vi "testMove.vi"() -> ()   [LabVIEW 2019]
uses:
  WSCbot_V3_Toolkit.lvlibp
panel:
  out "ENC (deg) 2":dbl[](array[numeric])
  in  "Enable?":bool=TRUE
  out "ENC (deg)":dbl[](array[numeric])
  in  "4xMotor(deg/s)":dbl[](array[numeric])=[0.0, 0.0, 0.0, 0.0]
  in  "Stop Button":bool
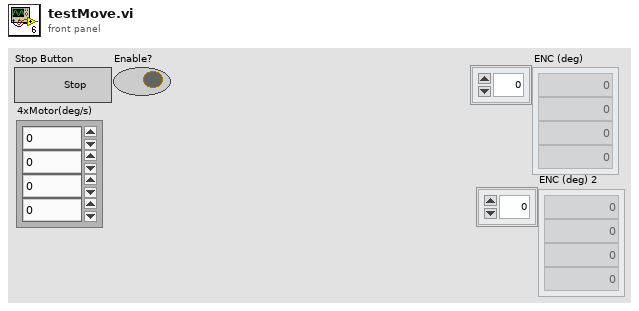
[diagram p1: front panel]
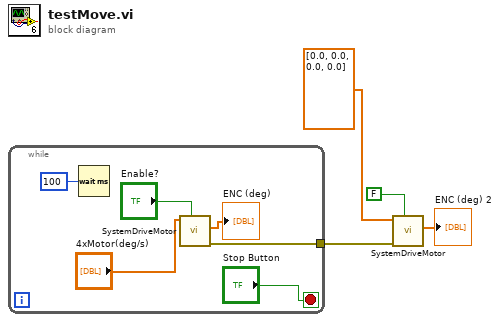
[diagram p0: block diagram]
diagram:
  n1 = while {
    tunnel: [w6] -> w4
    stop <- "Stop Button" stop-if-true
    n2 = Wait (ms)(milliseconds to wait=u32 100) -> ()  [unwired: 1 out]
    n3 = call "SystemDriveMotor.vi"("Enable?"="Enable?", "4xMotor(deg/s)"="4xMotor(deg/s)") -> ("error out"=w6:errorcluster, "ENC (deg)"=→"ENC (deg)":dbl[])  [unwired: 8 in]
  }
  n4 = call "SystemDriveMotor.vi"("Enable?"=FALSE ("Enable? 2"), "error in"=w4, "4xMotor(deg/s)"=dbl[] [0.0, 0.0, 0.0, 0.0]) -> ("ENC (deg)"=→"ENC (deg) 2":dbl[])  [unwired: 7 in, 1 out]
